vi "Get_arduino.vi"(11 "String":string) -> (2 "mean":dbl, 3 "Array":i32[](array[numeric]))   [LabVIEW 2013]
uses:
  <vilib>/Analysis/baseanly.llb/Mean (DBL).vi
  <vilib>/Analysis/NI_AALBase.lvlib
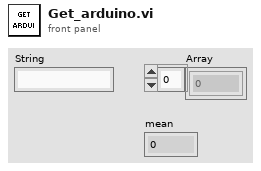
[diagram p1: front panel]
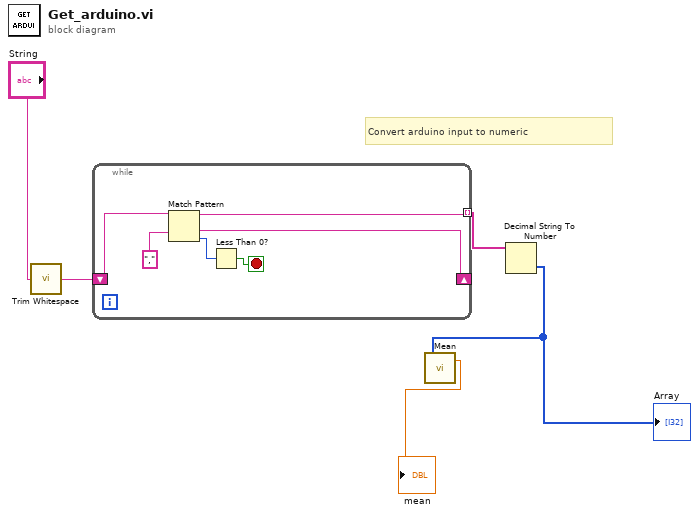
[diagram p0: block diagram]
diagram:
  # "Convert arduino input to numeric"
  n1 = call <vilib>:"Trim Whitespace.vi"("string"="String") -> ("trimmed string"=w3:string)  [unwired: 1 in]
  n2 = while {
    tunnel: [w8] -> w1 mode=indexing
    shift-right: [w9] -> _
    shift-left: w3 -> [w11]
    stop <- w6 stop-if-true
    n3 = Match Pattern(string=w11, regular expression=",") -> (before substring=w8:string, after substring=w9:string, offset past match=w7:i32)  [unwired: 2 out]
    n4 = Less Than 0?(x=w7) -> (x < 0?=w6:bool)
  }
  n5 = Decimal String To Number(string=w1) -> (number=w4:i32[])  [unwired: 1 in, 2 out]
  "Array" <- w4
  n6 = call-poly <vilib>:"Mean.vi"("X"=w4) -> ("mean"=→"mean":dbl)  [unwired: 1 out]
